vi "test Executable Path with Spaces.vi"(8 "error in":errorcluster) -> (0 "error out":errorcluster)   [LabVIEW 2024, in "serenial.io-ase.test.lvlib"]
uses:
  serenial.io-ase.test.lvlib
  <vilib>/addons/_JKI Toolkits/Caraya/classes/Assert/Assert.lvclass
  <vilib>/addons/_JKI Toolkits/Caraya/classes/Test/Test.lvclass
  serenial.io-ase/ase/ase.lvclass
  <vilib>/numeric/Random Number (Range) U64.vi
  <vilib>/addons/_JKI Toolkits/Caraya/classes/Assert/Assert Not Error.vi
  serenial.io-ase/ase/Start Call (Exe-Args).vi
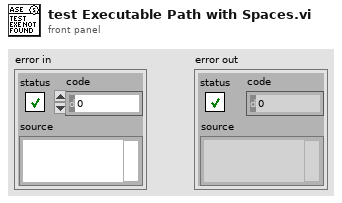
[diagram p1: front panel]
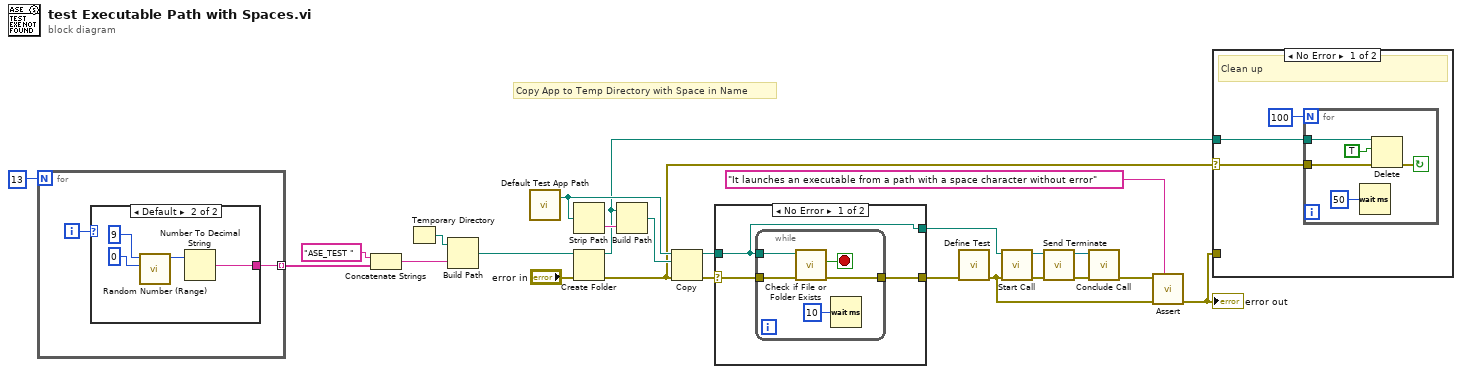
[diagram p0: block diagram]
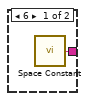
[diagram p4: hidden frame]
diagram:
  # "Copy App to Temp Directory with Space in Name"
  n1 = for {
    N: 13 -> [_]
    tunnel: [w26] -> w17 mode=indexing
    i -> [w25]
    n2 = case shown="Default" w25 {
      tunnel: [w27 w28] -> w26
      frame 6 {
        n3 = call <vilib>:"Space Constant.vi"() -> ("String"=w27:string)
      }
      frame Default {
        n4 = call-poly <vilib>:"Random Number (Range).vi"("lower bound (0)"=u64 0, "upper bound (100)"=u64 9) -> ("number"=w29:u64)  [unwired: 9 in]
        n5 = Number To Decimal String(number=w29) -> (decimal integer string=w28:string)  [unwired: 1 in]
      }
    }
  }
  n6 = Concatenate Strings("ASE_TEST ", w17) -> (w16:string)
  n7 = Temporary Directory() -> (w19:path)
  n8 = Build Path(base path=w19, name or relative path=w16) -> (appended path=w20:path)
  n9 = call "Default Test App Path.vi"() -> ("Exe Path With Extention"=w8:path)  [unwired: 2 in, 1 out]
  n10 = Strip Path(path=w8) -> (name=w9:string)  [unwired: 1 out]
  n11 = Create Folder(path (use dialog)=w20, error in="error in") -> (created path=w6:path, error out=w1:errorcluster)  [unwired: 1 in, 1 out]
  n12 = Build Path(base path=w6, name or relative path=w9) -> (appended path=w14:path)
  n13 = Copy(8:w1, 10:w14, 11:w8) -> (0:w2:errorcluster, 3:w5:path)  [unwired: 2 in, 1 out]
  n14 = case shown="No Error" w2 {
    selector: w2 -> [w34 w41]
    tunnel: [w33 w41] -> w3
    tunnel: [w32 w40] -> w4
    tunnel: w5 -> [w32 w40]
    frame No Error {
      n15 = while {
        tunnel: w34 -> [w39]
        tunnel: [w37] -> w33
        tunnel: w32 -> [w36]
        stop <- w38 stop-if-true
        n16 = call <vilib>:"Check if File or Folder Exists.vi"("error in (no error)"=w39, "path"=w36) -> ("error out"=w37:errorcluster, "file or folder exists?"=w38:bool)  [unwired: 7 in, 1 out]
        n17 = Wait (ms)(milliseconds to wait=u32 10) -> ()  [unwired: 1 out]
      }
    }
    frame Error {
    }
  }
  n18 = call <vilib>:"Define Test.vi"("error in (no error)"=w3) -> ("error out"=w10:errorcluster)  [unwired: 9 in, 1 out]
  n19 = call-poly "Start Call.vi"("error in"=w10, "Executable Path"=w4) -> ("error out"=w13:errorcluster, "New ASE Handle"=w23:refnum<class "ase.lvclass">)  [unwired: 8 in]
  n20 = call "Send Terminate.vi"("error in"=w13, "ASE Handle"=w23) -> ("error out"=w21:errorcluster, "ASE Handle Duplicate"=w22:refnum<class "ase.lvclass">)  [unwired: 7 in, 1 out]
  n21 = call "Conclude Call.vi"("error in"=w21, "ASE Handle"=w22) -> ("error out"=w11:errorcluster)  [unwired: 7 in, 2 out]
  n22 = call-poly <vilib>:"Assert.vi"("Label"="It launches an executable from a path with a space character without error", "error in (no error)"=w10, "Not Error?"=w11) -> ("error out"=w12:errorcluster)  [unwired: 7 in, 1 out]
  "error out" <- w12
  n23 = case shown="No Error" w1 {
    selector: w1 -> [w43 _]
    tunnel: w6 -> [w44 _]
    tunnel: w12 -> [_ _]
    frame No Error {
      # "Clean up"
      n24 = for {
        N: 100 -> [_]
        tunnel: w44 -> [w49]
        tunnel: w43 -> [w48]
        stop <- w45 continue-if-true
        n25 = Wait (ms)(milliseconds to wait=u32 50) -> ()  [unwired: 1 out]
        n26 = Delete(path (use dialog)=w49, entire hierarchy (F)=TRUE, error in=w48) -> (error out=w45:errorcluster)  [unwired: 2 in, 2 out]
      }
    }
    frame Error {
    }
  }
